vi "get.vi"(8 "error in (no error)":errorcluster, 10 "Name in":string, 11 "IStruct in":refnum<class "IStruct.lvclass">) -> (0 "error out":errorcluster, 2 "Field Value out":refnum<class "IBaseObject.lvclass">, 3 "IStruct out":refnum<class "IStruct.lvclass">)   [LabVIEW 2022 SP3, in "openDAQ.lvlib" / "daqCoreTypes.lvlib" / "IStruct.lvclass"]
uses:
  <instrlib>/openDAQ/Public/Classes/daqCoreTypes/IStruct/IStruct.lvclass
  <instrlib>/openDAQ/Public/Classes/daqCoreTypes/IStruct/IStruct.lvclass/IStruct.ctl
  <instrlib>/openDAQ/Public/Classes/IBaseObject/IBaseObject.lvclass
  <instrlib>/openDAQ/Binaries/Windows/x86/copendaq32.dll
  <instrlib>/openDAQ/Public/Classes/daqCoreTypes/IString/IString.lvclass
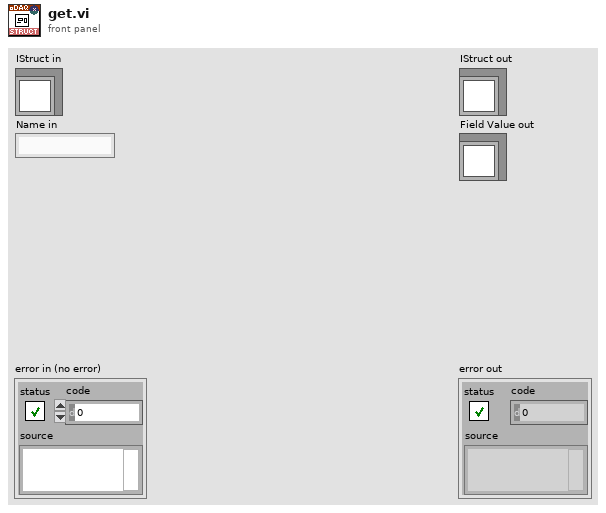
[diagram p1: front panel]
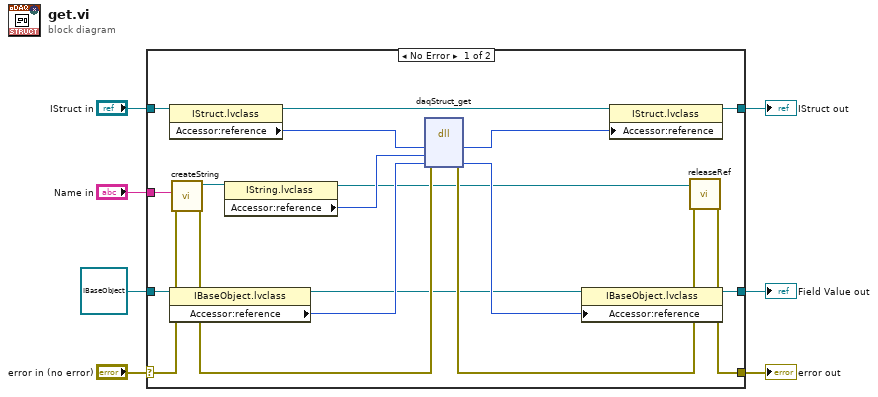
[diagram p0: block diagram]
diagram:
  n1 = case shown="No Error" "error in (no error)" {
    selector: "error in (no error)" -> [w15 w27]
    tunnel: [w10 w27] -> w6
    tunnel: [w20 w26] -> w4
    tunnel: "IStruct in" -> [w23 w26]
    tunnel: refnum<class "IBaseObject.lvclass"> refnum ("openDAQ.lvlib:IBaseObject.lvlib:IBaseObject.lvclass") -> [w18 _]
    tunnel: [w17 _] -> w2
    tunnel: "Name in" -> [w16 _]
    frame No Error {
      n2 = property class="IStruct.lvclass"(reference=w23) -> (reference out=w21:refnum<class "IStruct.lvclass">, "Accessor:reference"=w22:i64)  [unwired: 1 in, 1 out]
      n3 = property class="IBaseObject.lvclass"(reference=w18) -> (reference out=w8:refnum<class "IBaseObject.lvclass">, "Accessor:reference"=w24:i64)  [unwired: 1 in, 1 out]
      n4 = call <instrlib>:"createString.vi"("error in (no error)"=w15, "String"=w16) -> ("error out"=w14:errorcluster, "IString out"=w13:refnum<class "IString.lvclass">)  [unwired: 8 in]
      n5 = property class="IString.lvclass"(reference=w13) -> (reference out=w9:refnum<class "IString.lvclass">, "Accessor:reference"=w12:i64)  [unwired: 1 in, 1 out]
      n6 = dll-call lib="C:/Program Files (x86)/National Instruments/LabVIEW 2022/instr.lib/openDAQ/Binaries/Windows/x86/copendaq*.*" fn="daqStruct_get"(error in=w14, "struct"=w22, "name"=w12, "values"=w24) -> (error out=w11:errorcluster, "struct"=w19:i64, "values"=w25:i64)  [unwired: 4 in, 1 out]
      n7 = property class="IBaseObject.lvclass"(reference=w8, "Accessor:reference"=w25) -> (reference out=w17:refnum<class "IBaseObject.lvclass">)  [unwired: 1 in, 1 out]
      n8 = property class="IStruct.lvclass"(reference=w21, "Accessor:reference"=w19) -> (reference out=w20:refnum<class "IStruct.lvclass">)  [unwired: 1 in, 1 out]
      n9 = call-dynamic "releaseRef.vi"("error in (no error)"=w11, "IBaseObject in"=w9) -> ("error out"=w10:errorcluster)  [unwired: 9 in]
    }
    frame Error {
    }
  }
  "error out" <- w6
  "IStruct out" <- w4
  "Field Value out" <- w2
